vi "parse_config_string.vi"() -> ()   [LabVIEW 2013]
panel:
  out "Array":cluster{"name":string, "data":string}[](array[cluster])
  in  "String":string
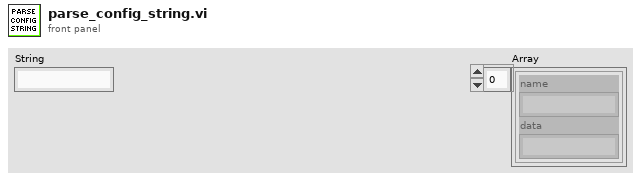
[diagram p1: front panel]
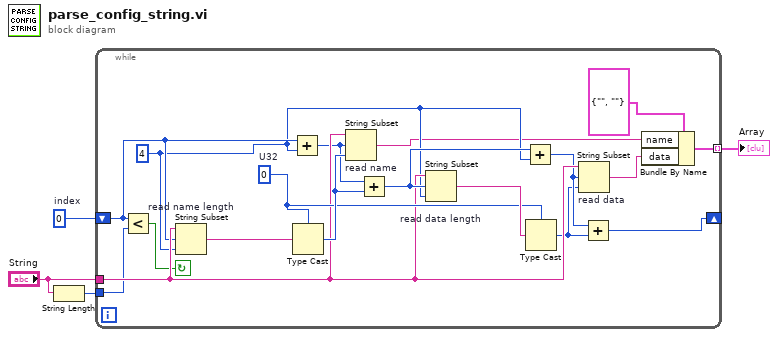
[diagram p0: block diagram]
diagram:
  w4 = u32 0  # index
  n1 = String Length(string="String") -> (length=w2:i32)
  n2 = while {
    shift-right: [w5] -> _
    shift-left: w4 -> [w14]
    tunnel: "String" -> [w17]
    tunnel: w2 -> [w16]
    tunnel: [w8] -> w1 mode=indexing
    stop <- w15 continue-if-true
    w19 = u32 0  # U32
    w12 = u32 4 ("length (rest)")
    n3 = Less?(x=w14, y=w16) -> (x < y?=w15:bool)
    n4 = String Subset "read name length"(string=w17, offset (0)=w14, length (rest)=w12) -> (substring=w22:string)
    n5 = Add(x=w14, y=w12) -> (x+y=w13:u32)
    n6 = Type Cast(type=w19, x=w22) -> (*(type *) &x=w21:u32)
    n7 = String Subset "read name"(string=w17, offset (0)=w13, length (rest)=w21) -> (substring=w10:string)
    n8 = Add(x=w13, y=w21) -> (x+y=w18:u32)
    n9 = String Subset "read data length"(string=w17, offset (0)=w18, length (rest)=w12) -> (substring=w20:string)
    n10 = Add(x=w18, y=w12) -> (x+y=w7:u32)
    n11 = Type Cast(type=w19, x=w20) -> (*(type *) &x=w6:u32)
    n12 = String Subset "read data"(string=w17, offset (0)=w7, length (rest)=w6) -> (substring=w9:string)
    n13 = Add(x=w7, y=w6) -> (x+y=w5:u32)
    n14 = Bundle By Name(cluster=cluster{"name":string, "data":string} {"name"="", "data"=""} ("input cluster"), "name"=w10, "data"=w9) -> (w8:cluster{"name":string, "data":string})
  }
  "Array" <- w1
